vi "Get Relay Names.vi"(8 "error in (no error)":errorcluster, 11 "SLSC Switch in":refnum<class "SLSC Switch.lvclass">) -> (0 "error out":errorcluster, 2 "Relay Names":string[](array[string]), 3 "SLSC Switch out":refnum<class "SLSC Switch.lvclass">)   [LabVIEW 2015, in "SLSC Switch.lvlib" / "SLSC Switch.lvclass"]
doc: "Retrurns a list of all relays available on the card."
uses:
  SLSC Switch.lvclass
  Switch Action Processor/Switch Action Processor.lvclass
  Relay/Relay.lvclass
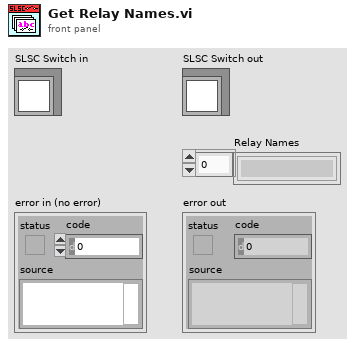
[diagram p1: front panel]
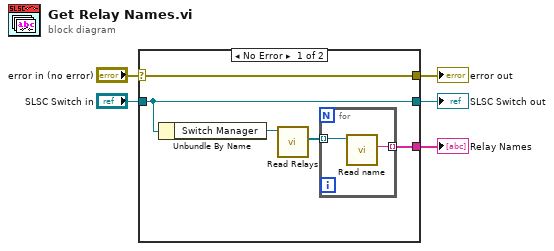
[diagram p0: block diagram]
diagram:
  n1 = case shown="No Error" "error in (no error)" {
    selector: "error in (no error)" -> [w10 w14]
    tunnel: [w10 w14] -> w4
    tunnel: [w9 _] -> w3
    tunnel: "SLSC Switch in" -> [w8 w13]
    tunnel: [w8 w13] -> w1
    frame No Error {
      n2 = Unbundle By Name(w8) -> ("Switch Manager"=w7:refnum<class "Switch Action Processor.lvclass">)
      n3 = call "Read Relays.vi"("Switch Action Processor in"=w7) -> ("Relays"=w6:refnum<class "Relay.lvclass">[])  [unwired: 9 in, 1 out]
      n4 = for {
        tunnel: w6 -> [w12] mode=indexing
        tunnel: [w11] -> w9 mode=indexing
        n5 = call "Read name.vi"("Relay in"=w12) -> ("name"=w11:string)  [unwired: 8 in, 2 out]
      }
    }
    frame Error {
    }
  }
  "error out" <- w4
  "Relay Names" <- w3
  "SLSC Switch out" <- w1
